vi "String.1D Str Array to LineFeed Delimited String.vi"(11 "Array":string[](array[string])) -> (3 "String":string)   [LabVIEW 2019]
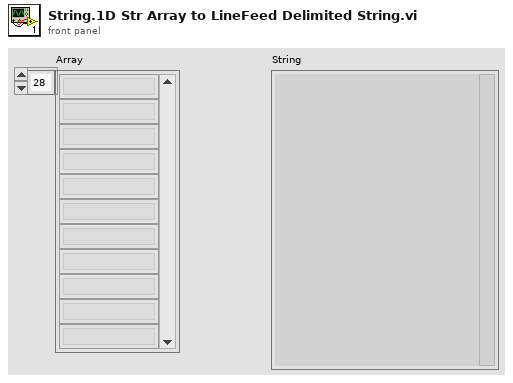
[diagram p1: front panel]
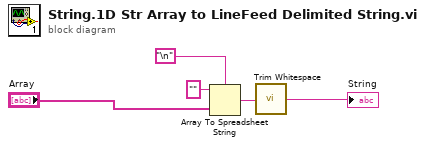
[diagram p0: block diagram]
diagram:
  n1 = Array To Spreadsheet String(delimiter (Tab)="\n", array="Array", 3:"" ("format string")) -> (spreadsheet string=w2:string)
  n2 = call <vilib>:"Trim Whitespace.vi"("string"=w2) -> ("trimmed string"=→"String":string)  [unwired: 1 in]
